vi "Fetch Waveforms.vi"(8 "error in (no error)":errorcluster, 11 "Scope Base in":refnum<class "Scope Base.lvclass">) -> (0 "error out":errorcluster, 3 "Scope Base out":refnum<class "Scope Base.lvclass">)   [LabVIEW 2023, in "Scope Base.lvlib" / "Scope Base.lvclass"]
uses:
  Scope Base.lvclass
  Scope Base.lvclass/Scope Base.ctl
  Interfaces/IConfigure Scope/IConfigure Scope.lvclass
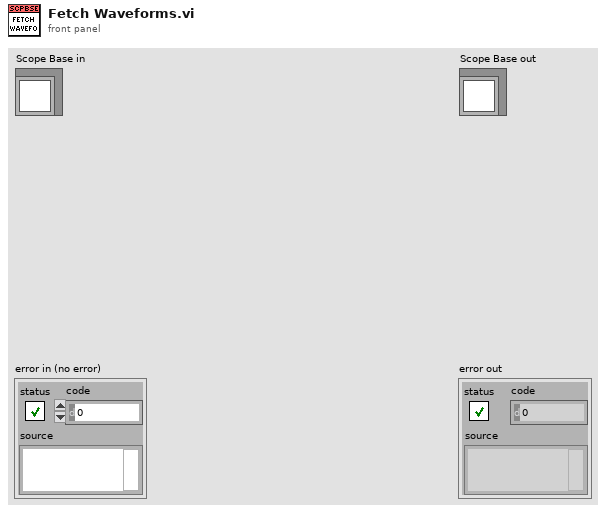
[diagram p1: front panel]
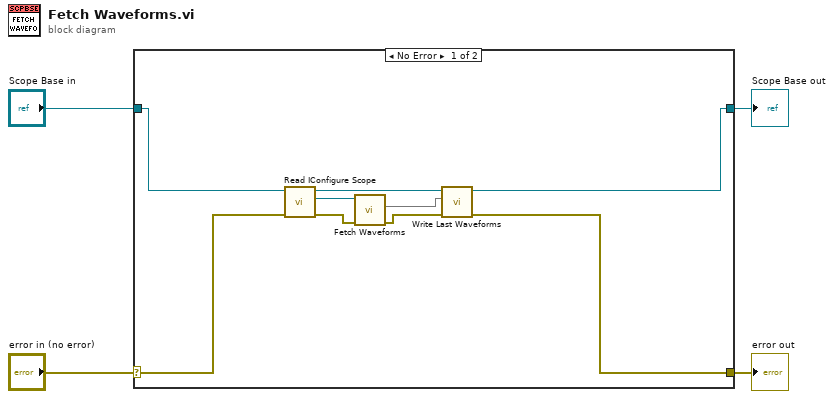
[diagram p0: block diagram]
diagram:
  n1 = case shown="No Error" "error in (no error)" {
    selector: "error in (no error)" -> [w13 w15]
    tunnel: [w8 w15] -> w3
    tunnel: [w6 w14] -> w1
    tunnel: "Scope Base in" -> [w12 w14]
    frame No Error {
      n2 = call "Read IConfigure Scope.vi"("error in (no error)"=w13, "Scope Base in"=w12) -> ("error out"=w10:errorcluster, "IConfigureScope"=w11:refnum<class "IConfigure Scope.lvclass">, "Scope Base out"=w7:refnum<class "Scope Base.lvclass">)  [unwired: 7 in]
      n3 = call-dynamic "Fetch Waveforms.vi"("error in (no error)"=w10, "IConfigure Scope in"=w11) -> ("error out"=w9:errorcluster, "Last Waveforms"=w5:map{u8, waveform(dbl)})  [unwired: 7 in, 1 out]
      n4 = call "Write Last Waveforms.vi"("error in (no error)"=w9, "Last Waveforms"=w5, "Scope Base in"=w7) -> ("error out"=w8:errorcluster, "Scope Base out"=w6:refnum<class "Scope Base.lvclass">)  [unwired: 7 in]
    }
    frame Error {
    }
  }
  "error out" <- w3
  "Scope Base out" <- w1
